vi "Initialize DAQ.vi"(8 "error in (no error)":errorcluster, 11 "DAQ Config Data In":T1) -> (0 "error out":errorcluster, 3 "DAQ Config Data Out":T1)   [LabVIEW 2020, in "Waveform Analog Output Engine.lvlib"]
doc: "Create and configure the analog output waveform task based on custom device settings"
uses:
  Waveform Analog Output Engine.lvlib
  DAQ Config Data.ctl
  <vilib>/DAQmx/create/channels.llb/DAQmx Create Channel (AO-Voltage-Basic).vi
  <vilib>/DAQmx/configure/timing.llb/DAQmx Timing (Sample Clock).vi
  Shared/Constants.vi
  <resource>/objmgr/daqmx.rc
  Shared/Waveform Analog Output Shared.lvlib
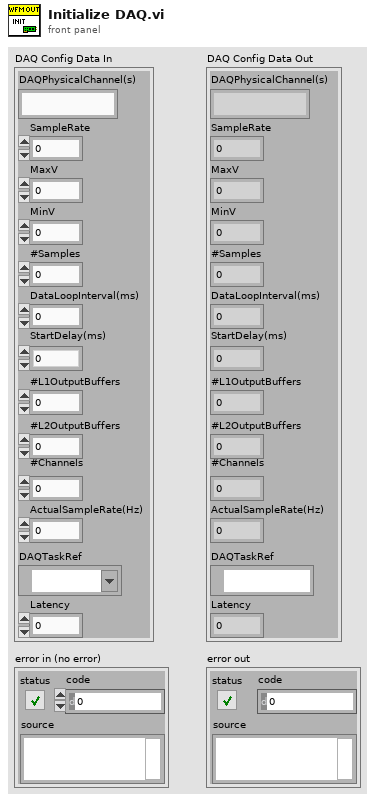
[diagram p1: front panel]
types:
  T1 = typedef "Waveform Analog Output Engine.lvlib/DAQ Config Data.ctl" = cluster{"DAQPhysicalChannel(s)":string, "SampleRate":dbl, "MaxV":dbl, "MinV":dbl, "#Samples":dbl, "DataLoopInterval(ms)":u32, "StartDelay(ms)":dbl, "#L1OutputBuffers":i32, "#L2OutputBuffers":i32, "#Channels":i32, "ActualSampleRate(Hz)":dbl, "DAQTaskRef":refnum<k21>, "Latency":dbl}
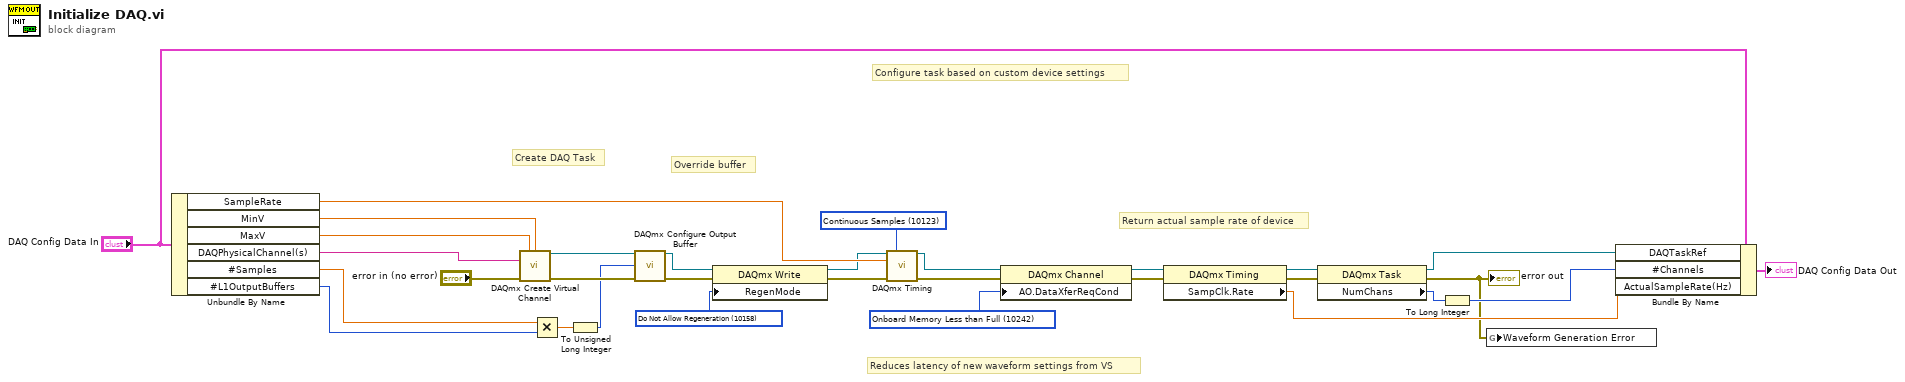
[diagram p0: block diagram]
diagram:
  w16 = 10123 items=["Finite Samples"=10178, "Continuous Samples"=10123, "Hardware Timed Single Point"=12522] ("sample mode")
  w17 = 10242 items=["Onboard Memory Empty"=10235, "Onboard Memory Half Full or Less"=10239, "Onboard Memory Less than Full"=10242] ("AO.DataXferReqCond")
  w25 = 10158 items=["Allow Regeneration"=10097, "Do Not Allow Regeneration"=10158] ("RegenMode")
  # "Reduces latency of new waveform settings from VS"
  # "Override buffer"
  # "Return actual sample rate of device"
  # "Configure task based on custom device settings"
  # "Create DAQ Task"
  n1 = Unbundle By Name("DAQ Config Data In") -> ("SampleRate"=w31:dbl, "MinV"=w23:dbl, "MaxV"=w24:dbl, "DAQPhysicalChannel(s)"=w12:string, "#Samples"=w10:dbl, "#L1OutputBuffers"=w8:i32)
  n2 = call-poly <vilib>:"DAQmx Create Virtual Channel.vi"("maximum value"=w24, "minimum value"=w23, "physical channels"=w12, "error in"="error in (no error)") -> ("task out"=w22:refnum<k21>, "error out"=w21:errorcluster)  [unwired: 10 in]
  n3 = Multiply(x=w10, y=w8) -> (x*y=w9:dbl)
  n4 = To Unsigned Long Integer(number=w9) -> (unsigned 32bit integer=w11:u32)
  n5 = call <vilib>:"DAQmx Configure Output Buffer.vi"("task/channels in"=w22, "buffer size (in samples per channel)"=w11, "error in"=w21) -> ("task out"=w20:refnum<k21>, "error out"=w19:errorcluster)  [unwired: 11 in]
  n6 = property class="DAQmx Write"(reference=w20, error in=w19, "RegenMode"=w25) -> (reference out=w27:refnum<k21>, error out=w26:errorcluster)
  n7 = call-poly <vilib>:"DAQmx Timing.vi"("task/channels in"=w27, "sample mode"=w16, "rate"=w31, "error in"=w26) -> ("task out"=w18:refnum<k21>, "error out"=w15:errorcluster)  [unwired: 10 in]
  n8 = property class="DAQmx Channel"(reference=w18, error in=w15, "AO.DataXferReqCond"=w17) -> (reference out=w14:refnum<k21>, error out=w13:errorcluster)
  n9 = property class="DAQmx Timing"(reference=w14, error in=w13) -> (reference out=w28:refnum<k21>, error out=w29:errorcluster, "SampClk.Rate"=w4:dbl)
  n10 = property class="DAQmx Task"(reference=w28, error in=w29) -> (reference out=w6:refnum<k21>, error out=w1:errorcluster, "NumChans"=w30:u32)
  "error out" <- w1
  n11 = To Long Integer(number=w30) -> (32bit integer=w5:i32)
  n12 = global write "Constants.vi" "Waveform Generation Error"(w1) -> ()
  n13 = Bundle By Name(cluster="DAQ Config Data In", "DAQTaskRef"=w6, "#Channels"=w5, "ActualSampleRate(Hz)"=w4) -> (→"DAQ Config Data Out":T1)
